vi "createStateChangedEvent.vi"(8 "error in (no error)":errorcluster, 11 "UserEvents in":refnum<class "UserEvents.lvclass">) -> (0 "error out":errorcluster, 3 "UserEvents out":refnum<class "UserEvents.lvclass">)   [LabVIEW 2016, in "UserEvents.lvclass"]
uses:
  UserEvents.lvclass
  Types/StateChangedEvent.ctl
  Types/Timestamp.ctl
  Types/SummaryStates.ctl
  Types/DetailedStates.ctl
  UserEvents.lvclass/UserEvents.ctl
  Types/M1M3SupportTypes.lvlib
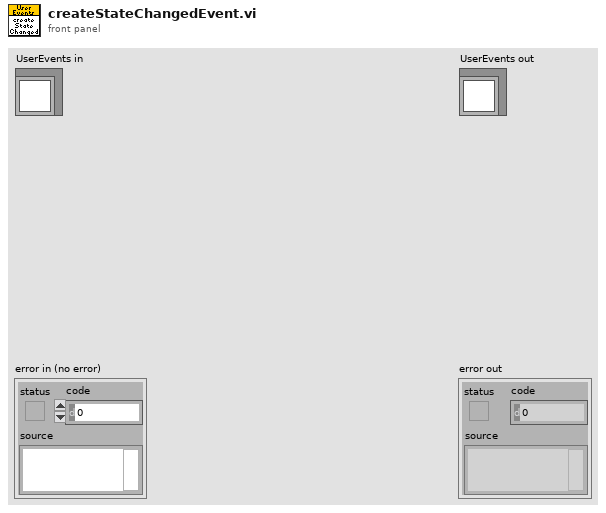
[diagram p1: front panel]
types:
  T1 = typedef "M1M3SupportTypes.lvlib/StateChangedEvent.ctl" = cluster{"Timestamp":T2, "SummaryStates":T3, "DetailedStates":T4}
  T2 = typedef "M1M3SupportTypes.lvlib/Timestamp.ctl" = dbl
  T3 = typedef "M1M3SupportTypes.lvlib/SummaryStates.ctl" = enum16{"OfflineState", "StandbyState", "DisabledState", "EnabledState", "FaultState"}
  T4 = typedef "M1M3SupportTypes.lvlib/DetailedStates.ctl" = enum16{"PublishOnlyState", "AvailableState", "StandbyState", "DisabledState", "EnabledState", "FaultState"}
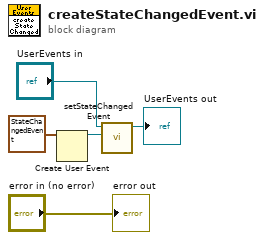
[diagram p0: block diagram]
diagram:
  n1 = Create User Event(user event datatype=T1 {"Timestamp"=0.0, "SummaryStates"=enum."OfflineState", "DetailedStates"=enum."PublishOnlyState"} ("StateChangedEvent")) -> (user event=w4:refnum<user-event>)  [unwired: 1 in, 1 out]
  n2 = call "setStateChangedEvent.vi"("StateChangedEvent"=w4, "UserEvents in"="UserEvents in") -> ("UserEvents out"=→"UserEvents out":refnum<class "UserEvents.lvclass">)  [unwired: 9 in]
  "error out" <- "error in (no error)"
